vi "Last Ack Created.vi"(10 "jettl":refnum<class "jettl.lvclass">, 11 "TEMPLATE jettl in":refnum<class "TEMPLATE jettl.lvclass">) -> (3 "TEMPLATE jettl out":refnum<class "TEMPLATE jettl.lvclass">)   [LabVIEW 2021, in "_Template.lvlib" / "Templates.lvlib" / "TEMPLATE jettl.lvlib" / "TEMPLATE jettl.lvclass"]
uses:
  TEMPLATE jettl.lvclass
  jettl/jettl/jettl/jettl.lvclass
  TEMPLATE jettl.lvclass/TEMPLATE jettl.ctl
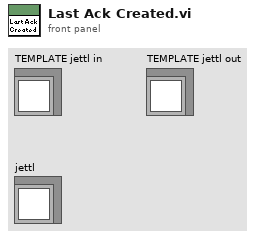
[diagram p1: front panel]
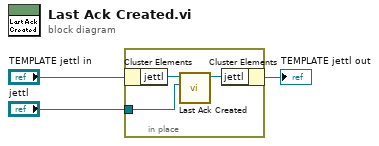
[diagram p0: block diagram]
diagram:
  n1 = in-place {
    in-place-border: "jettl" -> [w4]
    n2 = in-place-cluster #1("TEMPLATE jettl in") -> ("jettl"=w6:refnum<class "jettl.lvclass">)
    n3 = call-dynamic "Last Ack Created.vi"("jettl"=w4, "Last Ack Created in"=w6) -> ("Last Ack Created out"=w5:refnum<class "jettl.lvclass">)  [unwired: 9 in]
    n4 = in-place-cluster #1("jettl"=w5) -> (→"TEMPLATE jettl out":refnum<class "TEMPLATE jettl.lvclass">)
  }
